vi "Filter Name.vi"   [LabVIEW 2019]
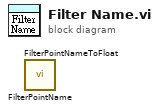
[diagram p0: block diagram]
diagram:
  n1 = call "FilterPointName.vi"() -> ()  [unwired: 5 in, 7 out]
  n2 = call "FilterPointNameToFloat.vi"() -> ()  [unwired: 5 in, 7 out]
